vi "Pre-Build Custom Action.vi"(10 "Variant":variant) -> (0 "error out":errorcluster)   [LabVIEW 2020]
uses:
  <vilib>/nisyscfg/Get Installed Components.vi
  <vilib>/Platform/browser.llb/Open URL in Default Browser (string).vi
  <vilib>/nisyscfg/nisyscfg.lvlib
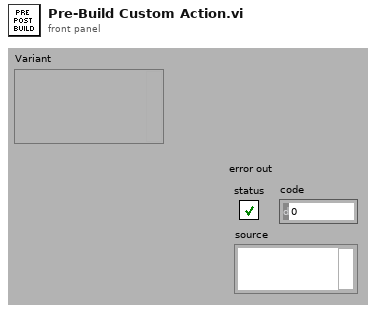
[diagram p1: front panel]
types:
  T1 = typedef "nisyscfg.lvlib/Software 1.2.ctl" = cluster{"title":string, "description":string, "ID":string, "version":string, "component type":T2}
  T2 = typedef "nisyscfg.lvlib/Component Type.ctl" = u32
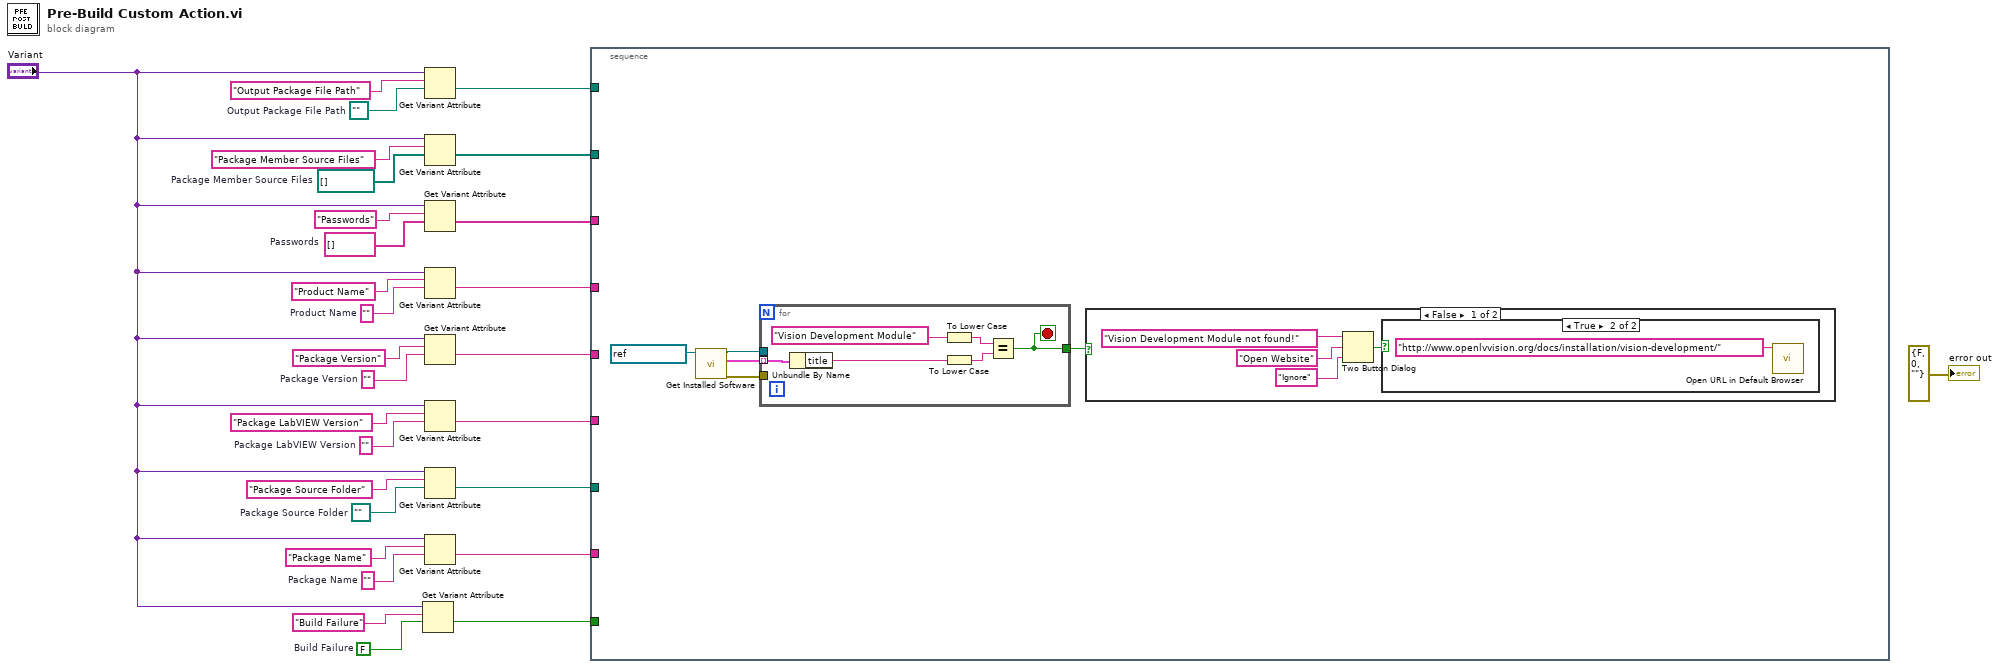
[diagram p0: block diagram]
diagram:
  w3 = FALSE  # Build Failure
  w13 = path ""  # Package Source Folder
  w14 = ""  # Package Name
  w17 = ""  # Package LabVIEW Version
  w19 = ""  # Package Version
  w21 = ""  # Product Name
  w24 = string[] []  # Passwords
  w26 = path[] []  # Package Member Source Files
  w28 = path ""  # Output Package File Path
  n1 = Get Variant Attribute(Variant="Variant", name="Build Failure", default value (empty Variant)=w3) -> (value=w1:bool)  [unwired: 1 in, 3 out]
  n2 = Get Variant Attribute(Variant="Variant", name="Output Package File Path", default value (empty Variant)=w28) -> (value=w12:path)  [unwired: 1 in, 3 out]
  n3 = Get Variant Attribute(Variant="Variant", name="Package Member Source Files", default value (empty Variant)=w26) -> (value=w11:path[])  [unwired: 1 in, 3 out]
  n4 = Get Variant Attribute(Variant="Variant", name="Passwords", default value (empty Variant)=w24) -> (value=w10:string[])  [unwired: 1 in, 3 out]
  n5 = Get Variant Attribute(Variant="Variant", name="Product Name", default value (empty Variant)=w21) -> (value=w9:string)  [unwired: 1 in, 3 out]
  n6 = Get Variant Attribute(Variant="Variant", name="Package Version", default value (empty Variant)=w19) -> (value=w8:string)  [unwired: 1 in, 3 out]
  n7 = Get Variant Attribute(Variant="Variant", name="Package LabVIEW Version", default value (empty Variant)=w17) -> (value=w7:string)  [unwired: 1 in, 3 out]
  n8 = Get Variant Attribute(Variant="Variant", name="Package Source Folder", default value (empty Variant)=w13) -> (value=w6:path)  [unwired: 1 in, 3 out]
  n9 = Get Variant Attribute(Variant="Variant", name="Package Name", default value (empty Variant)=w14) -> (value=w5:string)  [unwired: 1 in, 3 out]
  n10 = stacked-sequence {
    tunnel: w12 -> [_]
    tunnel: w11 -> [_]
    tunnel: w10 -> [_]
    tunnel: w9 -> [_]
    tunnel: w8 -> [_]
    tunnel: w7 -> [_]
    tunnel: w6 -> [_]
    tunnel: w5 -> [_]
    tunnel: w1 -> [_]
    frame #0 {
      n11 = call-poly <vilib>:"Get Installed Software.vi"("Session in"=refnum<k21> "localhost") -> ("error out"=w32:errorcluster, "Software Components"=w33:T1[], "Session out"=w31:refnum<k21>)  [unwired: 8 in]
      n12 = for {
        tunnel: w33 -> [w45] mode=indexing
        tunnel: w32 -> [_]
        tunnel: w31 -> [_]
        tunnel: [w40] -> w30
        stop <- w40 stop-if-true
        n13 = Unbundle By Name(w45) -> ("title"=w43:string)
        n14 = To Lower Case(string="Vision Development Module") -> (all lower case string=w42:string)
        n15 = To Lower Case(string=w43) -> (all lower case string=w41:string)
        n16 = Equal?(x=w42, y=w41) -> (x = y?=w40:bool)
      }
      n17 = case shown="False" w30 {
        frame False {
          n18 = Two Button Dialog(message="Vision Development Module not found!", 1:"Ignore" ("message"), 2:"Open Website" ("message")) -> (T button?=w35:bool)
          n19 = case shown="True" w35 {
            frame False {
            }
            frame True {
              n20 = call-poly <vilib>:"Open URL in Default Browser.vi"("URL"="http://www.openlvvision.org/docs/installation/vision-development/") -> ()  [unwired: 5 in, 2 out]
            }
          }
        }
        frame True {
        }
      }
    }
  }
  "error out" <- errorcluster {"status"=FALSE, "code"=0, "source"=""} ("error out")
